vi "Handle Command.vi"(8 "error in (no error)":errorcluster, 9 "Data":variant, 10 "Command":string, 11 "Instrument in":refnum<class "Instrument.lvclass">) -> (0 "error out":errorcluster, 1 "Processed Data":variant, 2 "Command":string, 3 "Instrument out":refnum<class "Instrument.lvclass">)   [LabVIEW 2019, in "Instrument.lvclass"]
doc: "Override to add additional commands supported by your Instrument."
uses:
  Instrument.lvclass
  Typedefs/Instrument.Commands--Enum.ctl
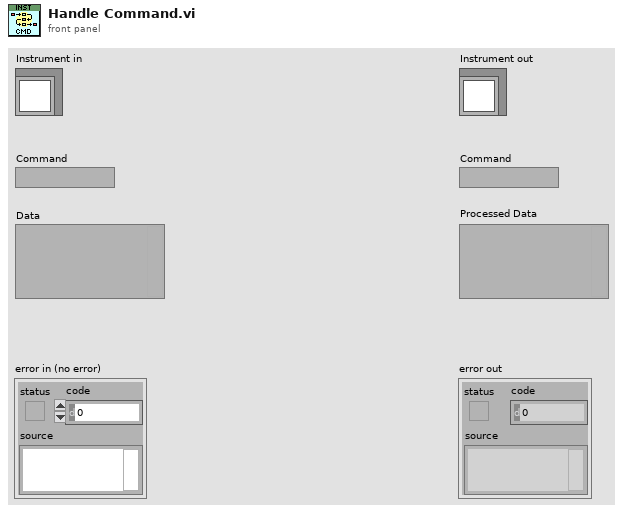
[diagram p1: front panel]
types:
  T1 = typedef "Instrument.lvclass/Instrument.Commands--Enum.ctl" = enum16{"ACK", "HELP", "setConfiguration", "setLogData", "getAll", "getAllData"}
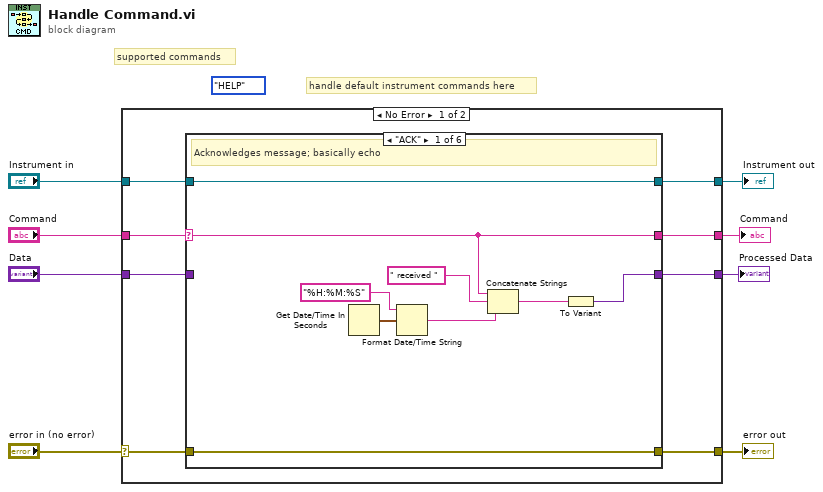
[diagram p0: block diagram]
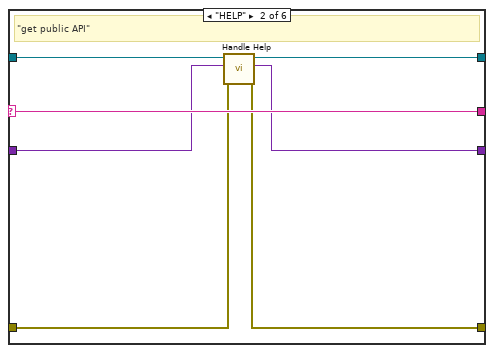
[diagram p2: hidden frame]
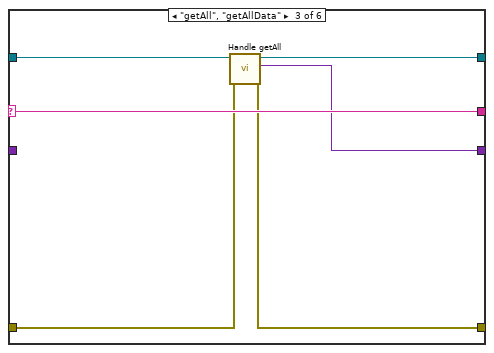
[diagram p3: hidden frame]
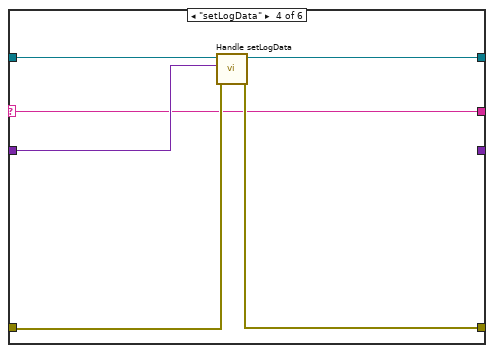
[diagram p4: hidden frame]
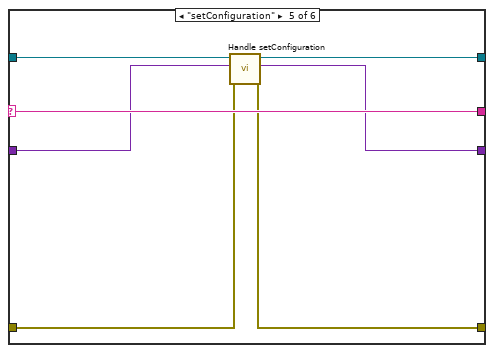
[diagram p5: hidden frame]
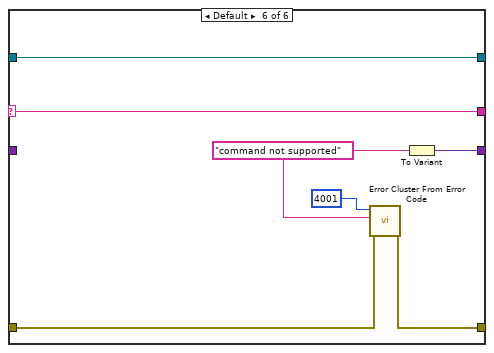
[diagram p6: hidden frame]
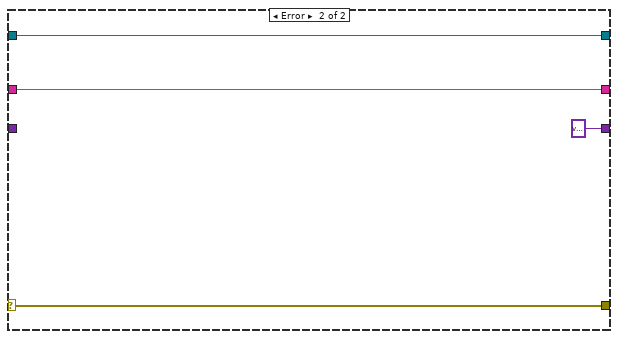
[diagram p7: hidden frame]
diagram:
  (unwired) Instrument.Commands--Enum."HELP" ("Commands")
  # "supported commands"
  # "handle default instrument commands here"
  n1 = case shown="No Error" "error in (no error)" {
    selector: "error in (no error)" -> [w13 w61]
    tunnel: [w12 w61] -> w7
    tunnel: [w15 w60] -> w5
    tunnel: "Instrument in" -> [w16 w60]
    tunnel: "Command" -> [w10 w58]
    tunnel: [w14 variant ("error message (\"\")")] -> w4
    tunnel: "Data" -> [w9 _]
    tunnel: [w11 w58] -> w1
    frame No Error {
      n2 = case shown="\"ACK\"" w10 {
        selector: w10 -> [w18 w30 w38 w39 w50 w55]
        tunnel: w16 -> [w25 w32 w35 w44 w47 w57]
        tunnel: [w25 w31 w34 w43 w46 w57] -> w15
        tunnel: [w20 w27 w33 _ w45 w56] -> w14
        tunnel: w13 -> [w22 w29 w37 w41 w49 w53]
        tunnel: [w22 w28 w36 w40 w48 w52] -> w12
        tunnel: [w18 w30 w38 w39 w50 w55] -> w11
        tunnel: w9 -> [_ w26 _ w42 w45 _]
        frame "ACK" {
          # "Acknowledges message; basically echo"
          n3 = Get Date/Time In Seconds() -> (seconds since 1Jan1904=w23:timestamp)
          n4 = Format Date/Time String(time format string (%c)="%H:%M:%S", seconds (now)=w23) -> (date/time string=w24:string)  [unwired: 1 in]
          n5 = Concatenate Strings(w18, " received " ("data"), w24) -> (w21:string)
          n6 = To Variant(anything=w21) -> (Variant=w20:variant)
        }
        frame "HELP" {
          # "\"get public API\""
          n7 = call-dynamic "Handle Help.vi"("error in (no error)"=w29, "Command"=w26, "Instrument in"=w32) -> ("error out"=w28:errorcluster, "Variant"=w27:variant, "Instrument out"=w31:refnum<class "Instrument.lvclass">)  [unwired: 6 in]
        }
        frame "getAll", "getAllData" {
          n8 = call-dynamic "Handle getAll.vi"("error in (no error)"=w37, "Instrument in"=w35) -> ("error out"=w36:errorcluster, "getAll"=w33:variant, "Instrument out"=w34:refnum<class "Instrument.lvclass">)  [unwired: 7 in]
        }
        frame "setLogData" {
          n9 = call-dynamic "Handle setLogData.vi"("error in (no error)"=w41, "LogData"=w42, "Instrument in"=w44) -> ("error out"=w40:errorcluster, "Instrument out"=w43:refnum<class "Instrument.lvclass">)  [unwired: 7 in]
        }
        frame "setConfiguration" {
          n10 = call-dynamic "Handle setConfiguration.vi"("error in (no error)"=w49, "setConfiguration"=w45, "Instrument in"=w47) -> ("error out"=w48:errorcluster, "Instrument out"=w46:refnum<class "Instrument.lvclass">)  [unwired: 7 in]
        }
        frame Default {
          w51 = "command not supported" ("error message (\"\")")
          n11 = call <vilib>:"Error Cluster From Error Code.vi"("error in (no error)"=w53, "error message (\"\")"=w51, "error code (0)"=4001) -> ("error out"=w52:errorcluster)  [unwired: 6 in]
          n12 = To Variant(anything=w51) -> (Variant=w56:variant)
        }
      }
    }
    frame Error {
    }
  }
  "error out" <- w7
  "Instrument out" <- w5
  "Processed Data" <- w4
  "Command" <- w1
